vi "Set Spliter Properties.vi"(0 "Display State In":T1, 1 "Height (Collapsed)":i32, 2 "Height (Expanded)":i32, 5 "index":i32, 9 "Container State":T4, 11 "error in (no error)":errorcluster, 12 "Expanded by Default":bool, 13 "Resizible":bool, 14 "Collapsable":bool) -> (4 "Display State Out":T1, 15 "error out":errorcluster)   [LabVIEW 2013, in "UI Panels.lvlib" / "Panels_XControl.xctl"]
uses:
  Panels_XControl.xctl
  <vilib>/_xctls/Container State.ctl
  State 1.ctl
  Controls/References/Panel_Refnums.ctl
  Controls/Panel_Command_Enum.ctl
  <vilib>/_xctls/XControlSupport.lvlib
panel:
  # "Add Controls & Indicators that form the parameters of the method here. Hook them to the connector pane. Do not delete the controls & indicators that are already hooked to the connector pane.\n \nTo setup the parameters  for this method, right click on this item in the Project Tree & select \"Configure Method...\"."
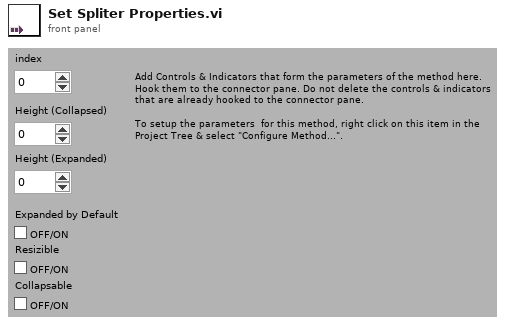
[diagram p1: front panel]
types:
  T1 = typedef "UI Panels.lvlib/Panels_XControl.xctl/State 1.ctl" = cluster{"Panels_Refnums_Array":T2[], "Panel_Command":cluster{"Operation":T3, "Data":variant}}
  T2 = typedef "UI Panels.lvlib/Panels_XControl.xctl/Panel_Refnums.ctl" = cluster{"VI Refnum":refnum<vi>, "Command":refnum<user-event>, "Visible":bool}
  T3 = typedef "UI Panels.lvlib/Panels_XControl.xctl/Panel_Command_Enum.ctl" = enum16{"Idle", "Remove & Stop", "Add Item", "Delete Item", "Delete All", "Insert into Subpanel", "Register Menu Events", "Update Value", "Remove from Subpanel", "Set Title", "Set Menu Items", "Insert SubPanel", "Set Splitter Position", "Set Splitter Properties", "Add Menu Items"}
  T4 = typedef "XControlSupport.lvlib/Container State.ctl" = cluster{"Indicator?":bool, "Run Mode?":bool, " Refnum":refnum<vi>}
  T5 = cluster{"index":i32, "Height (Collapsed)":i32, "Height (Expanded)":i32, "Expanded by Default":bool, "Collapsable":bool, "Resizible":bool}
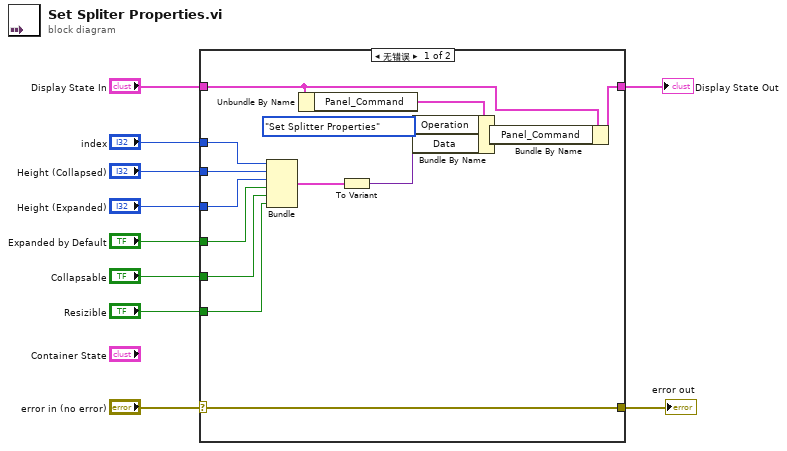
[diagram p0: block diagram]
diagram:
  n1 = case shown="无错误" "error in (no error)" {
    selector: "error in (no error)" -> [w11 w25]
    tunnel: [w20 w26] -> w10
    tunnel: "Display State In" -> [w19 w26]
    tunnel: "index" -> [w18 _]
    tunnel: "Height (Collapsed)" -> [w17 _]
    tunnel: "Height (Expanded)" -> [w16 _]
    tunnel: "Expanded by Default" -> [w15 _]
    tunnel: "Collapsable" -> [w14 _]
    tunnel: "Resizible" -> [w13 _]
    tunnel: [w11 w25] -> w1
    frame No Error {
      n2 = Bundle("index"=w18, "Height (Collapsed)"=w17, "Height (Expanded)"=w16, "Expanded by Default"=w15, "Collapsable"=w14, "Resizible"=w13) -> (w12:T5)  [unwired: 1 out]
      n3 = Unbundle By Name(w19) -> ("Panel_Command"=w21:cluster{"Operation":T3, "Data":variant})
      n4 = To Variant(anything=w12) -> (Variant=w23:variant)
      n5 = Bundle By Name(cluster=w21, "Operation"=Panel_Command_Enum."Set Splitter Properties", "Data"=w23) -> (w24:cluster{"Operation":T3, "Data":variant})
      n6 = Bundle By Name(cluster=w19, "Panel_Command"=w24) -> (w20:T1)
    }
    frame Error {
    }
  }
  "Display State Out" <- w10
  "error out" <- w1
